vi "Practica 3 Operaciones con Arrays.vi"() -> ()   [LabVIEW 2016]
panel:
  in  "Anterior":bool
  in  "Siguiente":bool
  out "Nombre Completo":string
  in  "Integrantes de Equipo":string[][](array[string])
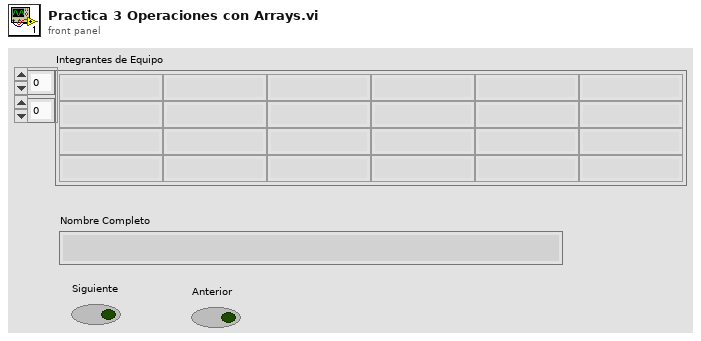
[diagram p1: front panel]
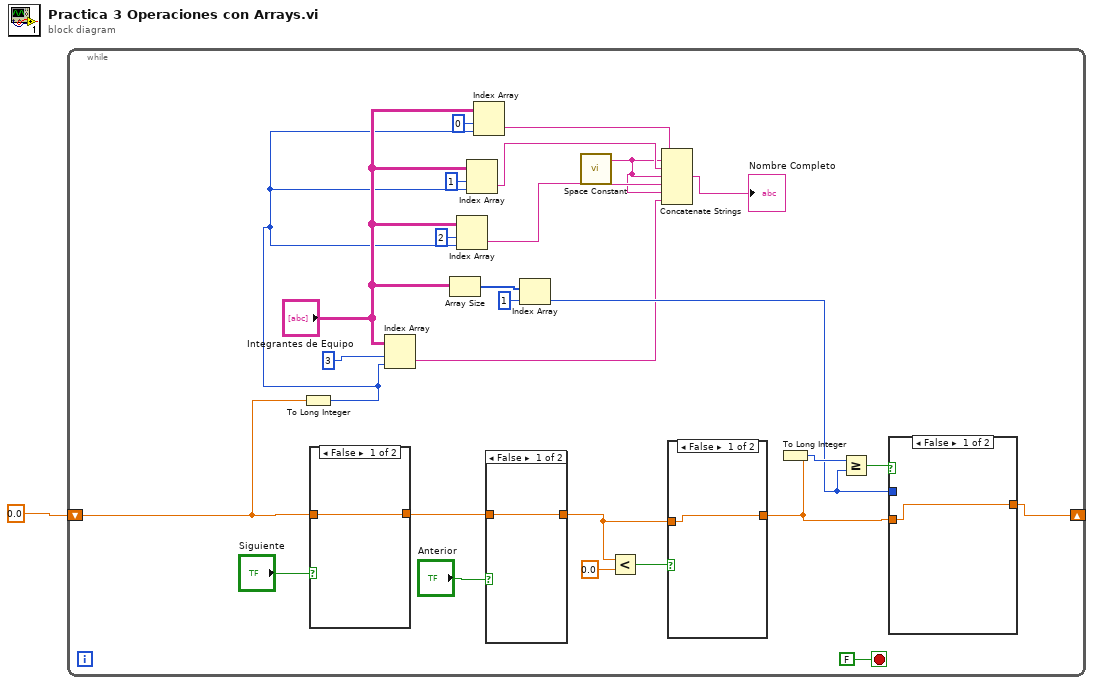
[diagram p0: block diagram]
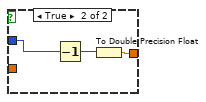
[diagram p2: hidden frame]
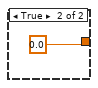
[diagram p3: hidden frame]
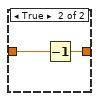
[diagram p4: hidden frame]
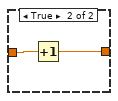
[diagram p5: hidden frame]
diagram:
  n1 = while {
    shift-right: [w16] -> _
    shift-left: 0.0 -> [w22]
    stop <- FALSE stop-if-true
    n2 = To Long Integer(number=w22) -> (32bit integer=w11:i32)
    n3 = case shown="False" "Siguiente" {
      tunnel: w22 -> [w38 w40]
      tunnel: [w38 w39] -> w26
      frame False {
      }
      frame True {
        n4 = Increment(x=w40) -> (x+1=w39:dbl)
      }
    }
    n5 = Index Array(array="Integrantes de Equipo", index (row)=3 ("disabled index (col)"), index (col)=w11) -> (element=w7:string)
    n6 = Array Size(array="Integrantes de Equipo") -> (size(s)=w20:i32[])
    n7 = Index Array(array="Integrantes de Equipo", index (row)=2 ("disabled index (row)"), index (col)=w11) -> (element=w6:string)
    n8 = Index Array(array="Integrantes de Equipo", index (row)=1 ("disabled index (row)"), index (col)=w11) -> (element=w4:string)
    n9 = Index Array(array="Integrantes de Equipo", index (row)=0 ("disabled index (row)"), index (col)=w11) -> (element=w3:string)
    n10 = case shown="False" "Anterior" {
      tunnel: w26 -> [w35 w37]
      tunnel: [w35 w36] -> w23
      frame False {
      }
      frame True {
        n11 = Decrement(x=w37) -> (x-1=w36:dbl)
      }
    }
    n12 = Index Array(array=w20, index=1) -> (element=w14:i32)
    n13 = call <vilib>:"Space Constant.vi"() -> ("String"=w2:string)
    n14 = Less?(x=w23, y=0.0) -> (x < y?=w24:bool)
    n15 = Concatenate Strings(w3, w2, w4, w2, w6, w2, w7) -> (→"Nombre Completo":string)
    n16 = case shown="False" w24 {
      tunnel: w23 -> [w33 _]
      tunnel: [w33 0.0] -> w17
      frame False {
      }
      frame True {
      }
    }
    n17 = To Long Integer(number=w17) -> (32bit integer=w15:i32)
    n18 = Greater Or Equal?(x=w15, y=w14) -> (x >= y?=w18:bool)
    n19 = case shown="False" w18 {
      tunnel: w17 -> [w29 _]
      tunnel: w14 -> [_ w31]
      tunnel: [w29 w32] -> w16
      frame False {
      }
      frame True {
        n20 = Decrement(x=w31) -> (x-1=w30:i32)
        n21 = To Double Precision Float(number=w30) -> (double precision float=w32:dbl)
      }
    }
  }
